vi "readDaq.vi"(8 "error in (no error)":errorcluster) -> (0 "error out":errorcluster, 3 "dataFifoFull":bool)   [LabVIEW 2018]
doc: "Read analog sensors and relays status from NI modules. Put this data into the <b>daqFIFO</b>."
uses:
  <vilib>/rvi/eio/common/nirviEmuTemplateMethod_errors.vi
  <vilib>/rvi/interface/RandomDataEmulation/niFpgaRandomDataHandleErrors.vi
  <vilib>/eio/EIONode/EIONode.xnode
  <vilib>/rvi/DataTransferAndStorage/Container/XNode/niFpgaContainer.xnode
  <vilib>/rvi/interface/RandomDataEmulation/nirviRandomDataFpgaReadWriteTemplate.vi
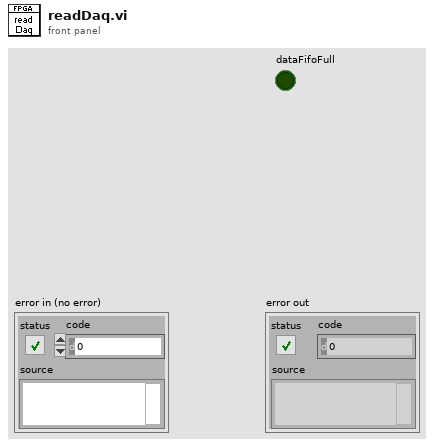
[diagram p1: front panel]
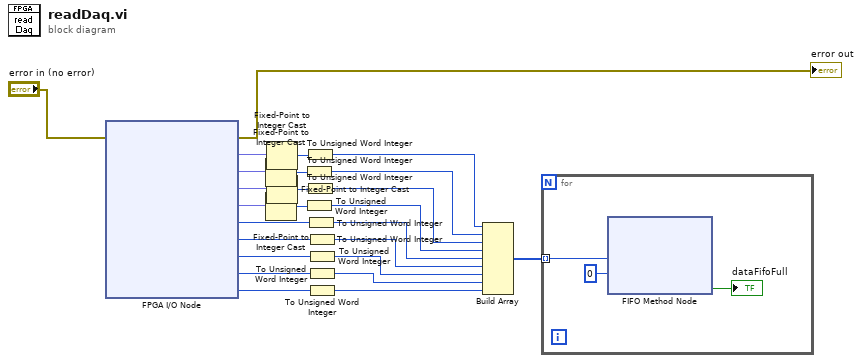
[diagram p0: block diagram]
diagram:
  n1 = xnode "FPGA I/O Node"("error in"="error in (no error)") -> ("error out"=→"error out":errorcluster, "ilcMotorCurrent"=w12:fxp<+/-,16,5>, "ilcCommCurrent"=w8:fxp<+/-,16,5>, "ilcMotorVoltage"=w5:fxp<+/-,16,7>, "ilcCommVoltage"=w4:fxp<+/-,16,7>, "Mod4/CH7:0"=w24:u8, "Mod5/DI7:0"=w23:u8, "Mod5/DI15:8"=w22:u8, "Mod5/DI23:16"=w21:u8, "Mod5/DI31:24"=w20:u8)  [unwired: 9 in, 9 out]
  n2 = Fixed-Point to Integer Cast(1:w8) -> (0:w9:i16)
  n3 = Fixed-Point to Integer Cast(1:w4) -> (0:w7:i16)
  n4 = Fixed-Point to Integer Cast(1:w12) -> (0:w11:i16)
  n5 = Fixed-Point to Integer Cast(1:w5) -> (0:w6:i16)
  n6 = To Unsigned Word Integer(number=w9) -> (unsigned 16bit integer=w3:u16)
  n7 = To Unsigned Word Integer(number=w7) -> (unsigned 16bit integer=w1:u16)
  n8 = To Unsigned Word Integer(number=w11) -> (unsigned 16bit integer=w10:u16)
  n9 = To Unsigned Word Integer(number=w6) -> (unsigned 16bit integer=w2:u16)
  n10 = To Unsigned Word Integer(number=w24) -> (unsigned 16bit integer=w19:u16)
  n11 = To Unsigned Word Integer(number=w23) -> (unsigned 16bit integer=w18:u16)
  n12 = To Unsigned Word Integer(number=w22) -> (unsigned 16bit integer=w17:u16)
  n13 = To Unsigned Word Integer(number=w21) -> (unsigned 16bit integer=w16:u16)
  n14 = To Unsigned Word Integer(number=w20) -> (unsigned 16bit integer=w15:u16)
  n15 = Build Array(w10, w3, w2, w1, w19, w18, w17, w16, w15) -> (w14:u16[])
  n16 = for {
    tunnel: w14 -> [w27] mode=indexing
    n17 = xnode ("FIFO Method Node")("Element"=w27, "Timeout"=0) -> ("Timed Out?"=→"dataFifoFull":bool)  [unwired: 1 in, 1 out]
  }
